vi "SYST_ERR_REP_SUNL.vi"(0 "VISA IN":refnum<visa-resource-name>, 5 "error in":errorcluster, 7 "Report":bool) -> (14 "VISA Out":refnum<visa-resource-name>, 19 "error out":errorcluster)   [LabVIEW 2018, in "PNA-X.lvlib"]
doc: "SYSTem:ERRor:REPort:SUNLeveled <bool> \n(Read-Write) Specifies whether or not to report Source Unleveled errors to the SCPI system error \nbuffer. \nParameters \n<bool> True (or 1) Report Source Unleveled Errors. Read errors from the system \nerror buffer using SYST:ERR? \nFalse (or 0) Do NOT report Source Unleveled Errors. \nExamples SYST:ERR:REP:SUNL 1 \nsystem:error:report:sunleveled true \nQuery Syntax SYSTem:ERRor:REPort:UNLeveled? \nDefault False"
uses:
  PNA-X.lvlib
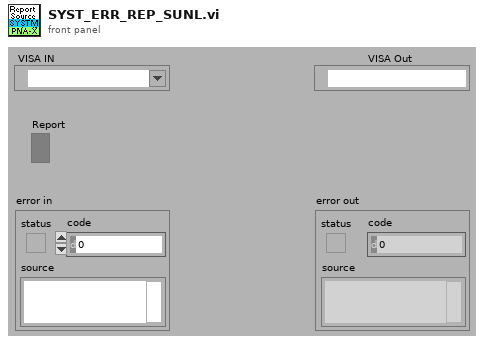
[diagram p1: front panel]
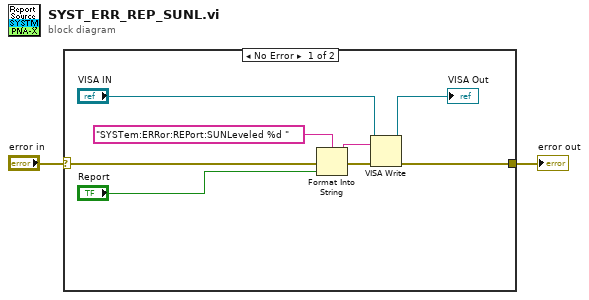
[diagram p0: block diagram]
diagram:
  n1 = case shown="No Error" "error in" {
    selector: "error in" -> [w10 w11]
    tunnel: [w5 w11] -> w1
    frame No Error {
      n2 = Format Into String(format string="SYSTem:ERRor:REPort:SUNLeveled %d " ("Cmdline"), error in=w10, "Report") -> (resulting string=w8:string, error out=w9:errorcluster)  [unwired: 1 in]
      n3 = VISA Write(VISA resource name="VISA IN", write buffer=w8, error in (no error)=w9) -> (VISA resource name out=→"VISA Out":refnum<visa-resource-name>, error out=w5:errorcluster)  [unwired: 1 out]
    }
    frame Error {
    }
  }
  "error out" <- w1
